vi "PH_DeformableMirror.Init.vi"(0 "VI in":refnum<vi>, 5 "error in (no error)":errorcluster) -> (14 "VI out":refnum<vi>, 19 "error out":errorcluster)   [LabVIEW 2014, in "PH_DeformableMirror.lvlib"]
uses:
  PH_DeformableMirror.lvlib
  CSlibraries-extern/shs/packages/dmdriver/DMirrorBase/DMirrorBase.lvclass
  CSlibraries-extern/shs/packages/dmdriver/DMirrorUSB/DMirrorUSB.lvclass
  PH_Basics/PH_Common/PH_Common.lvlib
  CS_Core/CSSystem/CSSystemLib/CSSystemLib.lvlib
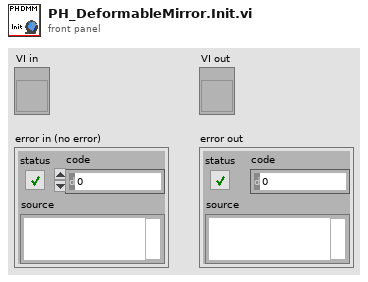
[diagram p1: front panel]
types:
  T1 = typedef "PH_DeformableMirror.lvlib/PH_DeformableMirror.i attribute.ctl" = cluster{"DMirror.lvlib:DMirrorBase.lvclass":refnum<class "DMirrorBase.lvclass">, "Device error":errorcluster, "GUI Refs":cluster{"Delete":refnum<vi>, "Device Error":refnum<vi>, "HV on":refnum<vi>, "Channel":refnum<vi>, "Voltage":refnum<vi>, "Channel Voltages":refnum<vi>}}
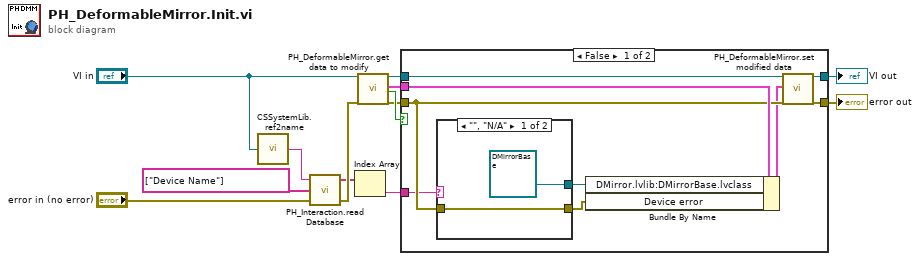
[diagram p0: block diagram]
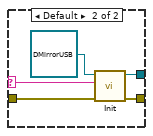
[diagram p2: hidden frame]
diagram:
  n1 = call "CSSystemLib.ref2name.vi"("obj refnum"="VI in") -> ("name"=w3:string)
  n2 = call "PH_Interaction.read Database.vi"("error in (no error)"="error in (no error)", "Strings to search for"=string[] ["Device Name"], "DB Entry to read"=w3) -> ("error out"=w10:errorcluster, "Values"=w1:string[])  [unwired: 1 in]
  n3 = Index Array(array=w1) -> (element=w11:string)  [unwired: 1 in]
  n4 = call "PH_DeformableMirror.get data to modify.vi"("i ref in"="VI in", "error in (no error)"=w10) -> ("i ref out"=w8:refnum<vi>, "i attribute"=w6:T1, "timed out"=w9:bool, "error out"=w7:errorcluster)  [unwired: 14 in]
  n5 = case shown="False" w9 {
    tunnel: w6 -> [w21 _]
    tunnel: w7 -> [w20 w30]
    tunnel: [w17 w30] -> w12
    tunnel: w8 -> [w22 w31]
    tunnel: [w16 w31] -> w13
    tunnel: w11 -> [w15 _]
    frame False {
      n6 = case shown="\"\", \"N/A\"" w15 {
        selector: w15 -> [_ w25]
        tunnel: w20 -> [w24 w28]
        tunnel: [w24 w27] -> w19
        tunnel: [refnum<class "DMirrorBase.lvclass"> refnum ("DMirror.lvlib:DMirrorBase.lvclass") w26] -> w14
        frame "", "N/A" {
        }
        frame Default {
          n7 = call-dynamic "Init.vi"("error in (no error)"=w28, "device name (dev1)"=w25, "DMirrorUSB in"=refnum<class "DMirrorUSB.lvclass"> refnum ("DMirror.lvlib:DMirrorUSB.lvclass")) -> ("error out"=w27:errorcluster, "DMirrorUSB out"=w26:refnum<class "DMirrorUSB.lvclass">)  [unwired: 7 in]
        }
      }
      n8 = Bundle By Name(cluster=w21, "DMirror.lvlib:DMirrorBase.lvclass"=w14, "Device error"=w19) -> (w18:T1)
      n9 = call "PH_DeformableMirror.set modified data.vi"("i ref in"=w22, "i attribute"=w18, "error in (no error)"=w20) -> ("i ref out"=w16:refnum<vi>, "error out"=w17:errorcluster)  [unwired: 15 in]
    }
    frame True {
    }
  }
  "VI out" <- w13
  "error out" <- w12
